vi "Lock Control in The Right.vi"(6 "offset":cluster{"x":i32, "y":i32}, 8 "error in (no error)":errorcluster, 11 "TabControl in":refnum<vi>) -> (0 "error out":errorcluster)   [LabVIEW 2017]
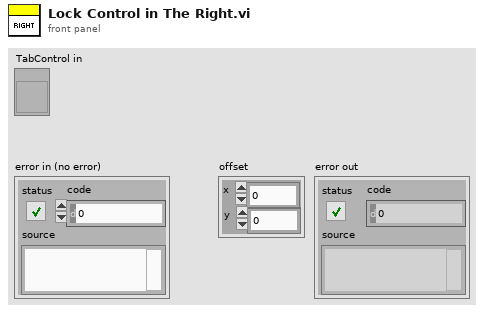
[diagram p1: front panel]
types:
  T1 = typedef "LVBoundsTypeDef.ctl" = cluster{"Width":u32, "Height":u32}
  T2 = typedef "LVPositionTypeDef.ctl" = cluster{"Left":i32, "Top":i32}
  T3 = cluster{"left":i16, "top":i16, "right":i16, "bottom":i16}
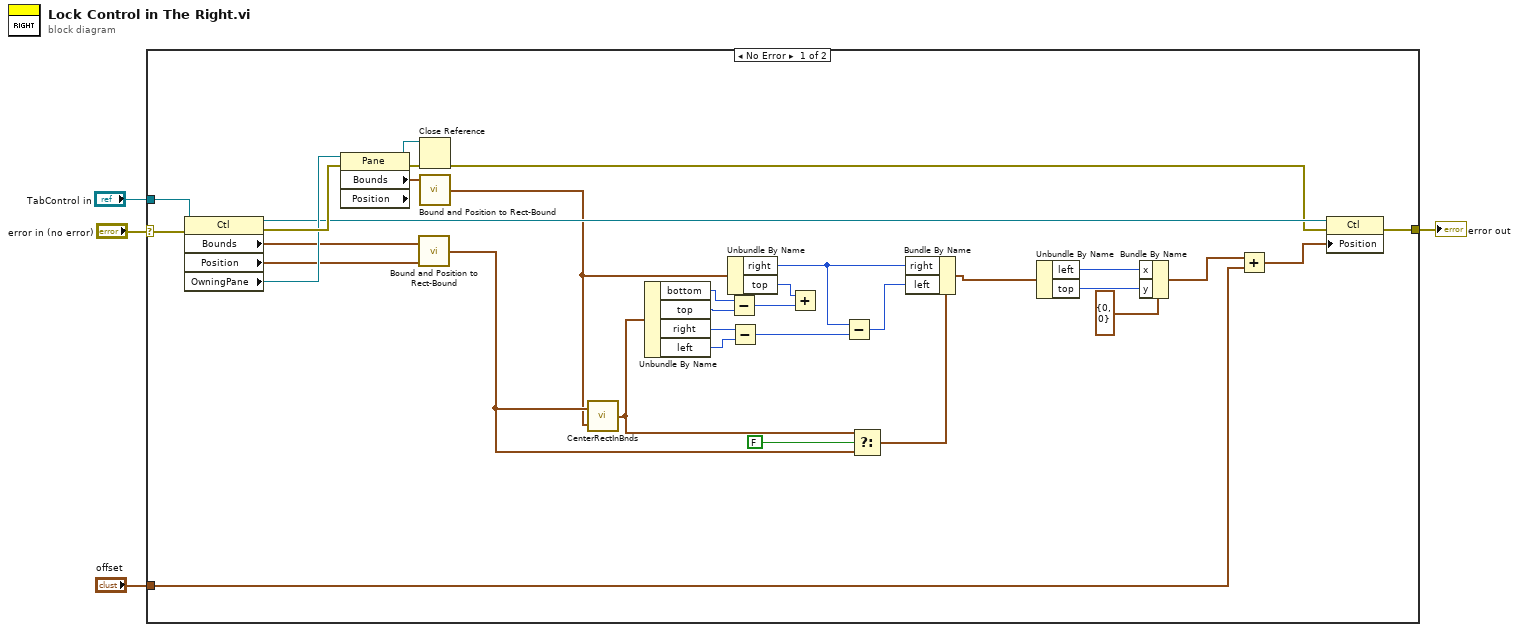
[diagram p0: block diagram]
diagram:
  n1 = case shown="No Error" "error in (no error)" {
    selector: "error in (no error)" -> [w26 w38]
    tunnel: "TabControl in" -> [w28 _]
    tunnel: [w27 w38] -> w3
    tunnel: "offset" -> [w21 _]
    frame No Error {
      n2 = property on="Property Node" class="Ctl"(reference=w28, error in=w26) -> (reference out=w34:refnum<vi>, error out=w36:errorcluster, "Bounds"=w29:T1, "Position"=w30:T2, "OwningPane"=w35:refnum<vi>)
      n3 = property on="Property Node" class="Pane" props=["Bounds", "Position"](reference=w35, error in=w36) -> (reference out=w24:refnum<vi>, error out=w37:errorcluster, "Bounds"=w31:T1)  [unwired: 1 out]
      n4 = call "Bound and Position to Rect-Bound.vi"("Position"=w30, "Bounds"=w29) -> ("Rect Bound"=w33:T3)  [unwired: 3 in]
      n5 = Close Reference(reference=w24, error in (no error)=w37) -> (error out=w25:errorcluster)
      n6 = call "Bound and Position to Rect-Bound.vi"("Bounds"=w31) -> ("Rect Bound"=w32:T3)  [unwired: 4 in]
      n7 = call <vilib>:"CenterRectInBnds.vi"("bounds"=w32, "rect"=w33) -> ("centered rect"=w17:T3)
      n8 = Unbundle By Name(w17) -> ("bottom"=w8:i16, "top"=w9:i16, "right"=w12:i16, "left"=w13:i16)
      n9 = Unbundle By Name(w32) -> ("right"=w14:i16, "top"=w11:i16)
      n10 = Subtract(x=w8, y=w9) -> (x-y=w10:i16)
      n11 = Subtract(x=w12, y=w13) -> (x-y=w15:i16)
      n12 = Add(x=w11, y=w10) -> ()  [unwired: 1 out]
      n13 = Subtract(x=w14, y=w15) -> (x-y=w16:i16)
      n14 = Select(t=w17, s=FALSE ("centered? (F)"), f=w33) -> (s? t:f=w18:T3)
      n15 = Bundle By Name(cluster=w18, "right"=w14, "left"=w16) -> (w23:T3)
      n16 = Unbundle By Name(w23) -> ("left"=w6:i16, "top"=w7:i16)
      n17 = Bundle By Name(cluster=cluster{"x":i32, "y":i32} {"x"=0, "y"=0} ("Point"), "x"=w6, "y"=w7) -> (w22:cluster{"x":i32, "y":i32})
      n18 = Add(x=w22, y=w21) -> (x+y=w20:cluster{"x":i32, "y":i32})
      n19 = property on="Property Node" class="Ctl"(reference=w34, error in=w25, "Position"=w20) -> (error out=w27:errorcluster)  [unwired: 1 out]
    }
    frame Error {
    }
  }
  "error out" <- w3
